vi "hasAttributeByType.vi"(7 "Attribute Type":refnum<class "Attribute.lvclass">, 8 "error in (no error)":errorcluster, 11 "SMO in":refnum<class "SMO.lvclass">) -> (0 "error out":errorcluster, 1 "found":bool, 3 "SMO out":refnum<class "SMO.lvclass">)   [LabVIEW 2021, in "smo.lvlib" / "SMO.lvclass"]
uses:
  SMO.lvclass
  Support/Attribute/Attribute.lvclass
  Support/Attribute/Attribute.lvclass/Attribute.ctl
  SMO.lvclass/SMO.ctl
  Private/ReftoDVR--SMO.vi
  <vilib>/Utility/LVClass/Get LV Class Name.vi
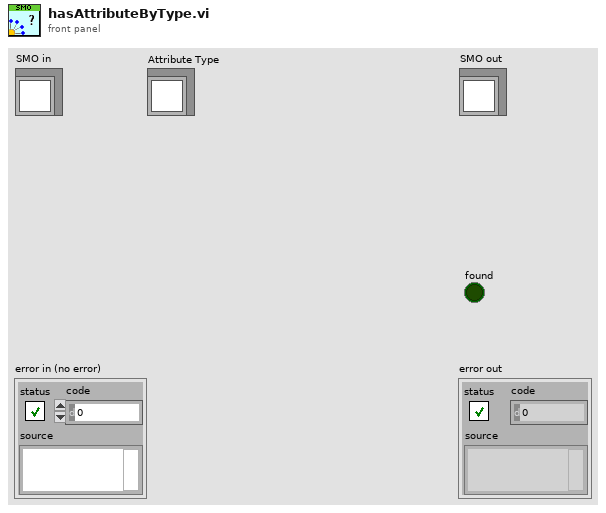
[diagram p1: front panel]
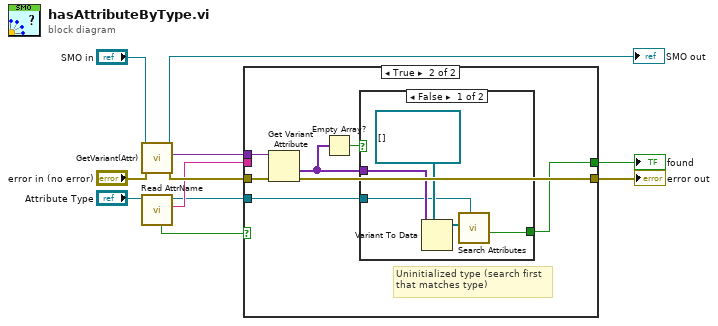
[diagram p0: block diagram]
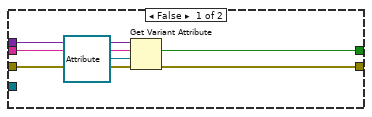
[diagram p2: hidden frame]
diagram:
  n1 = call "GetVariant(Attr).vi"("error in (no error)"="error in (no error)", "SMO in"="SMO in") -> ("error out"=w10:errorcluster, "[Attributes]"=w8:variant, "SMO out"=→"SMO out":refnum<class "SMO.lvclass">)  [unwired: 7 in]
  n2 = call "Read AttrName.vi"("Attribute in"="Attribute Type") -> ("Attribute Name"=w5:string, "Attribute out"=w4:refnum<class "Attribute.lvclass">, "unnamed"=w1:bool)  [unwired: 8 in]
  n3 = case shown="True" w1 {
    tunnel: w10 -> [w17 w23]
    tunnel: [w16 w22] -> w9
    tunnel: w8 -> [w15 w24]
    tunnel: [w14 w20] -> w7
    tunnel: w5 -> [w12 _]
    tunnel: w4 -> [_ w21]
    frame False {
      n4 = Get Variant Attribute(Variant=w15, name=w12, default value (empty Variant)=refnum<class "Attribute.lvclass"> refnum ("Attribute.lvclass"), error in=w17) -> (found=w14:bool, error out=w16:errorcluster)  [unwired: 2 out]
    }
    frame True {
      # "Uninitialized type (search first\nthat matches type)"
      n5 = Get Variant Attribute(Variant=w24, error in=w23) -> (values=w19:variant[], error out=w22:errorcluster)  [unwired: 2 in, 2 out]
      n6 = Empty Array?(array=w19) -> (empty?=w18:bool)
      n7 = case shown="False" w18 {
        tunnel: w21 -> [w25 _]
        tunnel: [w27 _] -> w20
        tunnel: w19 -> [w28 _]
        frame False {
          n8 = Variant To Data(type=refnum<class "Attribute.lvclass">[] [] ("[Attributes]"), Variant=w28) -> (data=w26:refnum<class "Attribute.lvclass">[])  [unwired: 1 in, 1 out]
          n9 = call "Search Attributes.vi"("Attribute type"=w25, "[Attributes]"=w26) -> ("found"=w27:bool)  [unwired: 8 in, 1 out]
        }
        frame True {
        }
      }
    }
  }
  "error out" <- w9
  "found" <- w7
